vi "onHttpPut (File).vi"(8 "error in":errorcluster, 10 "httpRequest":refnum<class "httpRequest.lvclass">, 11 "http-method in":refnum<class "REST Client.lvclass">) -> (0 "error out":errorcluster, 2 "httpResponse":refnum<class "httpResponse.lvclass">, 3 "http-method out":refnum<class "REST Client.lvclass">)   [LabVIEW 2020, in "REST Client.lvlib" / "REST Client.lvclass"]
uses:
  REST Client.lvclass
  REST Client.lvclass/REST Client.ctl
  http-client-pkg/httpClient/httpClient.lvclass
  http-client-pkg/httpRequest/httpRequest.lvclass
  http-client-pkg/httpResponse/httpResponse.lvclass
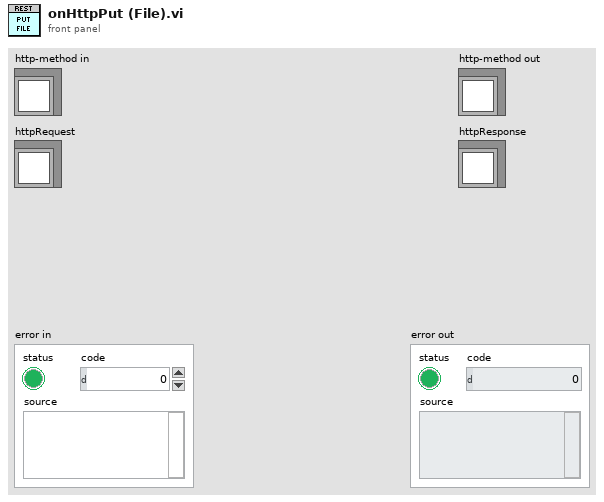
[diagram p1: front panel]
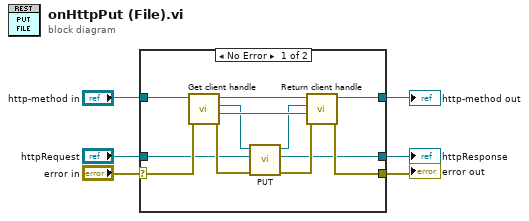
[diagram p0: block diagram]
diagram:
  n1 = case shown="No Error" "error in" {
    selector: "error in" -> [w14 w20]
    tunnel: [w11 w20] -> w1
    tunnel: [w12 w19] -> w5
    tunnel: "http-method in" -> [w13 w19]
    tunnel: "httpRequest" -> [w9 _]
    tunnel: [w10 _] -> w2
    frame No Error {
      n2 = call "Get client handle.vi"("error in (no error)"=w14, "REST Client in"=w13) -> ("error out"=w16:errorcluster, "Headers dup"=w17:refnum<class "httpHeaders.lvclass">, "http-client"=w8:refnum<class "httpClient.lvclass">, "REST Client out"=w18:refnum<class "REST Client.lvclass">)  [unwired: 6 in]
      n3 = call "PUT.vi"("error in"=w16, "httpRequest"=w9, "http-client in"=w8) -> ("error out"=w15:errorcluster, "httpResponse"=w10:refnum<class "httpResponse.lvclass">, "http-client out"=w7:refnum<class "httpClient.lvclass">)  [unwired: 6 in]
      n4 = call "Return client handle.vi"("error in (no error)"=w15, "Headers"=w17, "http-client"=w7, "REST Client in"=w18) -> ("error out"=w11:errorcluster, "REST Client out"=w12:refnum<class "REST Client.lvclass">)  [unwired: 6 in]
    }
    frame Error {
    }
  }
  "error out" <- w1
  "http-method out" <- w5
  "httpResponse" <- w2
